vi "Pass Args as Cluster.vi"() -> ()   [LabVIEW 2020]
uses:
  G-Embedded-Python-Interpreter-Toolkit/G-Embedded-Python-Interpreter-Toolkit.lvlib
  <vilib>/addons/_JKI Toolkits/Caraya/classes/Test/Test.lvclass
panel:
  out "error out":errorcluster
  in  "error in (no error)":errorcluster
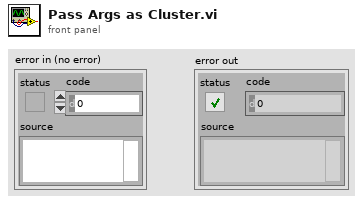
[diagram p1: front panel]
types:
  T1 = typedef "G-Embedded-Python-Interpreter-Toolkit.lvlib/Python Object Reference.ctl" = refnum<k1>
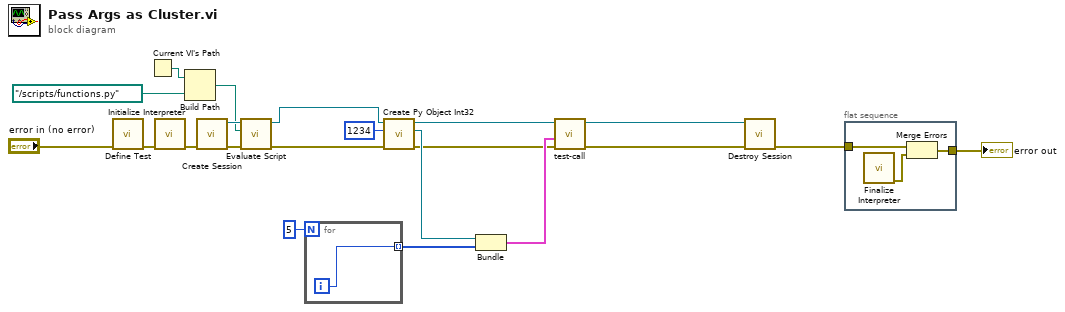
[diagram p0: block diagram]
diagram:
  n1 = call <vilib>:"Define Test.vi"("error in (no error)"="error in (no error)") -> ("error out"=w21:errorcluster)  [unwired: 10 in]
  n2 = Current VI's Path() -> (path=w16:path)
  n3 = call "Initialize Interpreter.vi"("error in (no error)"=w21) -> ("error out"=w18:errorcluster)  [unwired: 9 in, 1 out]
  n4 = Build Path(base path=w16, name or relative path=path "../scripts/functions.py" ("Path")) -> (appended path=w14:path)
  n5 = call "Create Session.vi"("error in (no error)"=w18) -> ("error out"=w13:errorcluster, "Session Handle"=w17:refnum<data-value>)  [unwired: 9 in]
  n6 = call "Evaluate Script.vi"("error in (no error)"=w13, "Script File Path"=w14, "Session Handle in"=w17) -> ("error out"=w10:errorcluster, "Session Handle out"=w11:refnum<data-value>)  [unwired: 7 in]
  n7 = for {
    N: 5 -> [_]
    tunnel: [w22] -> w7 mode=indexing
    i -> [w22]
  }
  n8 = call "Create Py Object Int32.vi"("error in (no error)"=w10, "Value"=1234, "Session Handle in"=w11) -> ("error out"=w3:errorcluster, "Python Object Refnum"=w8:T1, "Session Handle out"=w5:refnum<data-value>)  [unwired: 6 in]
  n9 = Bundle("Python Object Refnum"=w8, w7) -> (w4:cluster{"Python Object Refnum":T1, i32[]})  [unwired: 1 in]
  n10 = call "test-call.vi"("error in (no error)"=w3, "Arguments"=w4, "Data Value Reference in"=w5) -> ("error out"=w2:errorcluster, "Data Value Reference out"=w1:refnum<data-value>)  [unwired: 6 in, 1 out]
  n11 = call "Destroy Session.vi"("error in (no error)"=w2, "Session Handle"=w1) -> ("error out"=w12:errorcluster)  [unwired: 9 in]
  n12 = flat-sequence {
    tunnel: w12 -> [w25]
    tunnel: [w23] -> w19
    frame #0 {
      n13 = call "Finalize Interpreter.vi"() -> ("error out"=w24:errorcluster)  [unwired: 11 in]
      n14 = Merge Errors(w25, w24) -> (w23:errorcluster)
    }
  }
  "error out" <- w19
